vi "SW_Save_proc_data_to_TDMS.vi"(6 "TTL IO and Key in":string[][](array[string]), 7 "Processed animal coordinates and speed":T1, 8 "error in (no error)":errorcluster, 9 "HW timestamp and delta in":u32[][](array[numeric]), 10 "SW timestamp in":dbl[](array[numeric]), 11 "TDMS file ref. in":refnum<k34>) -> (0 "error out":errorcluster)   [LabVIEW 2018, in "Tracker.lvlib"]
uses:
  Tracker.lvlib
  Controls/CTL_Animal_Coordinates_and_Speed_(arr).ctl
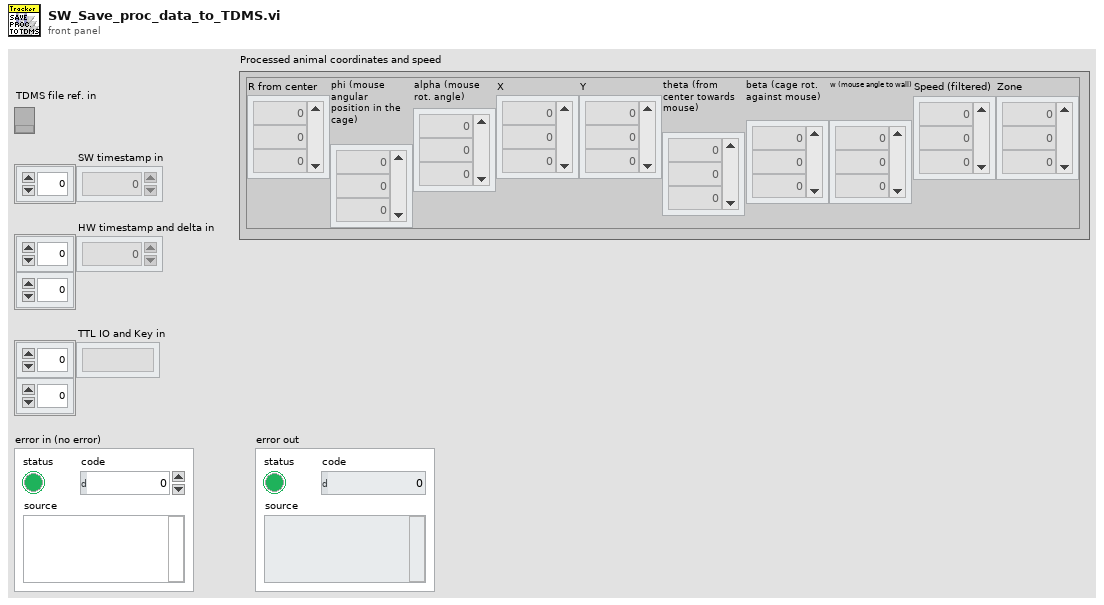
[diagram p1: front panel]
types:
  T1 = typedef "Tracker.lvlib/CTL_Animal_Coordinates_and_Speed_(arr).ctl" = cluster{"R from center":dbl[], "phi (mouse angular position in the cage)":dbl[], "alpha (mouse rot. angle)":dbl[], "X":dbl[], "Y":dbl[], "theta (from center towards mouse)":dbl[], "beta (cage rot. against mouse)":dbl[], "w (mouse angle to wall)":dbl[], "Speed (filtered)":dbl[], "Zone":i8[]}
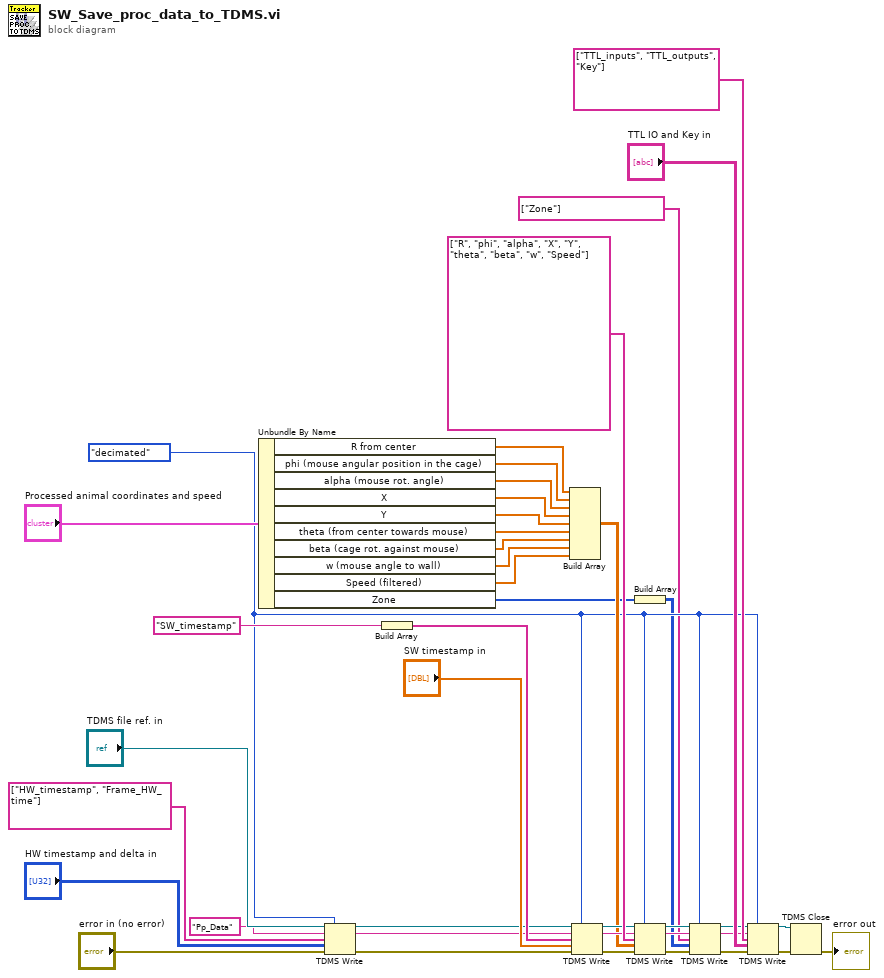
[diagram p0: block diagram]
diagram:
  w4 = enum16{"decimated", "interleaved"}."decimated" ("data layout (0:decimated)")
  n1 = Unbundle By Name("Processed animal coordinates and speed") -> ("R from center"=w21:dbl[], "phi (mouse angular position in the cage)"=w20:dbl[], "alpha (mouse rot. angle)"=w14:dbl[], "X"=w16:dbl[], "Y"=w15:dbl[], "theta (from center towards mouse)"=w19:dbl[], "beta (cage rot. against mouse)"=w18:dbl[], "w (mouse angle to wall)"=w17:dbl[], "Speed (filtered)"=w13:dbl[], "Zone"=w2:i8[])
  n2 = TDMS Write(0:"TDMS file ref. in", 1:w4, 5:"Pp_Data" ("group name in (Untitled)"), 7:string[] ["HW_timestamp", "Frame_HW_time"] ("appended array"), 9:"HW timestamp and delta in", 11:"error in (no error)") -> (4:w24:refnum<k34>, 6:w26:string, 15:w25:errorcluster)  [unwired: 1 out]
  n3 = Build Array("SW_timestamp" ("channel name(s) in (Untitled)")) -> (w28:string[])
  n4 = Build Array(w21, w20, w14, w16, w15, w19, w18, w17, w13) -> (w11:dbl[][])
  n5 = TDMS Write(0:w24, 1:w4, 5:w26, 7:w28, 9:"SW timestamp in", 11:w25) -> (4:w33:refnum<k34>, 6:w34:string, 15:w32:errorcluster)  [unwired: 1 out]
  n6 = Build Array(w2) -> (w1:i8[][])
  n7 = TDMS Write(0:w33, 1:w4, 5:w34, 7:string[] ["R", "phi", "alpha", "X", "Y", "theta", "beta", "w", "Speed"] ("appended array"), 9:w11, 11:w32) -> (4:w5:refnum<k34>, 6:w6:string, 15:w7:errorcluster)  [unwired: 1 out]
  n8 = TDMS Write(0:w5, 1:w4, 5:w6, 7:string[] ["Zone"] ("channel name(s) in (Untitled)"), 9:w1, 11:w7) -> (4:w10:refnum<k34>, 6:w9:string, 15:w8:errorcluster)  [unwired: 1 out]
  n9 = TDMS Write(0:w10, 1:w4, 5:w9, 7:string[] ["TTL_inputs", "TTL_outputs", "Key"] ("channel name(s) in (Untitled)"), 9:"TTL IO and Key in", 11:w8) -> (4:w36:refnum<k34>, 15:w37:errorcluster)  [unwired: 2 out]
  n10 = TDMS Close(8:w37, 11:w36) -> (0:→"error out":errorcluster)  [unwired: 1 out]
